vi "Update Next Button Visibility.vi"(8 "error in (no error)":errorcluster, 11 "Test Channel Model in":refnum<class "Test Channel Model.lvclass">) -> (0 "error out":errorcluster, 3 "Test Channel Model out":refnum<class "Test Channel Model.lvclass">)   [LabVIEW 2013, in "Test Channel Model.lvlib" / "Test Channel Model.lvclass"]
uses:
  Test Channel Model.lvclass
  Test Channel Model.lvclass/Test Channel Model.ctl
  <vilib>/ActorFrameworkMVC/View Observer/View Registry/View Registry.lvclass/View Registry.ctl
  Test Channel Model Messages/Abstract Test Channel Next Button Visibility Msg/Abstract Test Channel Next Button Visibility Msg.lvclass
  <vilib>/ActorFrameworkMVC/View Observer/Data Message/Data Message.lvclass
  <vilib>/ActorFrameworkMVC/View Observer/View Registry/View Registry.lvclass
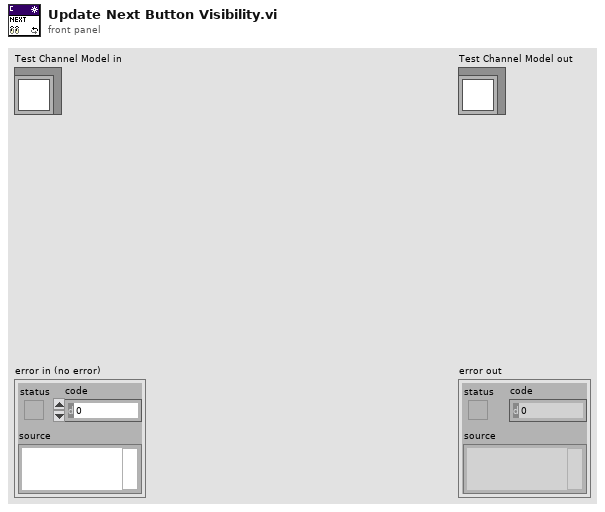
[diagram p1: front panel]
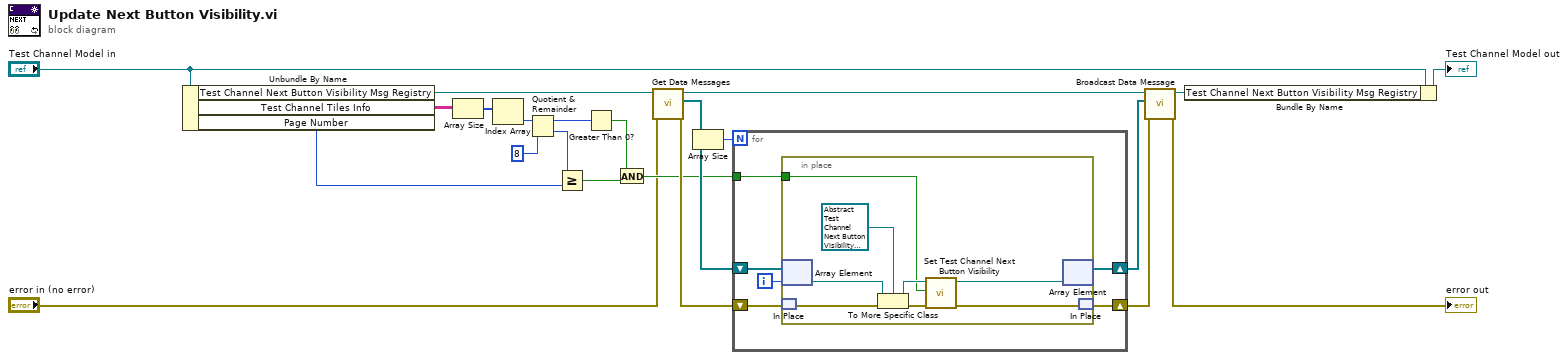
[diagram p0: block diagram]
diagram:
  n1 = Unbundle By Name("Test Channel Model in") -> ("Test Channel Next Button Visibility Msg Registry"=w22:refnum<class "View Registry.lvclass">, "Test Channel Tiles Info"=w9:string[][], "Page Number"=w6:i32)
  n2 = Array Size(array=w9) -> (size(s)=w8:i32[])
  n3 = Index Array(array=w8) -> (element=w7:i32)  [unwired: 1 in]
  n4 = Quotient & Remainder(x=w7, y=8) -> (x-y*floor(x/y)=w13:i32, floor(x/y)=w12:i32)
  n5 = Greater Or Equal?(x=w12, y=w6) -> (x >= y?=w15:bool)
  n6 = Greater Than 0?(x=w13) -> (x > 0?=w11:bool)
  n7 = And(x=w11, y=w15) -> (x .and. y?=w10:bool)
  n8 = call <vilib>:"Get Data Messages.vi"("error in (no error)"="error in (no error)", "View Registry in"=w22) -> ("error out"=w18:errorcluster, "Data Messages"=w19:refnum<class "Data Message.lvclass">[], "View Registry out"=w21:refnum<class "View Registry.lvclass">)  [unwired: 7 in]
  n9 = Array Size(array=w19) -> (size(s)=w20:i32)
  n10 = for {
    N: w20 -> [_]
    shift-right: [w27] -> w17
    shift-left: w19 -> [w28]
    shift-right: [w25] -> w16
    shift-left: w18 -> [w26]
    tunnel: w10 -> [w23]
    i -> [w24]
    n11 = in-place {
      in-place-border: w23 -> [w29]
      n12 = in-place-array #1(w28, w24) -> (w34:refnum<class "Data Message.lvclass">)
      n13 = in-place-match #2(w26) -> (w36:errorcluster)
      n14 = To More Specific Class(target class=refnum<class "Abstract Test Channel Next Button Visibility Msg.lvclass"> refnum ("Test Channel Model.lvlib:Abstract Test Channel Next Button Visibility Msg.lvclass"), reference=w34, error in=w36) -> (specific class reference=w30:refnum<class "Abstract Test Channel Next Button Visibility Msg.lvclass">, error out=w33:errorcluster)
      n15 = call "Set Test Channel Next Button Visibility.vi"("error in (no error)"=w33, "Test Channel Next Button Visibility"=w29, "Abstract Test Channel Next Button Visibility Msg in"=w30) -> ("error out"=w32:errorcluster, "Abstract Test Channel Next Button Visibility Msg out"=w31:refnum<class "Abstract Test Channel Next Button Visibility Msg.lvclass">)  [unwired: 7 in]
      n16 = in-place-array #1(w31) -> (w27:refnum<class "Data Message.lvclass">[])  [unwired: 1 out]
      n17 = in-place-match #2(w32) -> (w25:errorcluster)
    }
  }
  n18 = call <vilib>:"Broadcast Data Message.vi"("error in (no error)"=w16, "Data Messages"=w17, "View Registry in"=w21) -> ("error out"=→"error out":errorcluster, "View Registry out"=w5:refnum<class "View Registry.lvclass">)  [unwired: 7 in]
  n19 = Bundle By Name(cluster="Test Channel Model in", "Test Channel Next Button Visibility Msg Registry"=w5) -> (→"Test Channel Model out":refnum<class "Test Channel Model.lvclass">)
